vi "Untitled 3.vi"() -> ()   [LabVIEW 2016]
panel:
  out "channel name(s) in (Untitled)":string[](array[string])=["C0", "C1", "C2", "C3", "C4", "C5", "C6", "C7", "C8", "PCR-KW-A", "PCR-KW-B", "PCR-KW-C", "C12", "C13", "C14", "C15", "C16", "C17", "C18", "C19", "C20", "C21", "C22", "", "", ""]
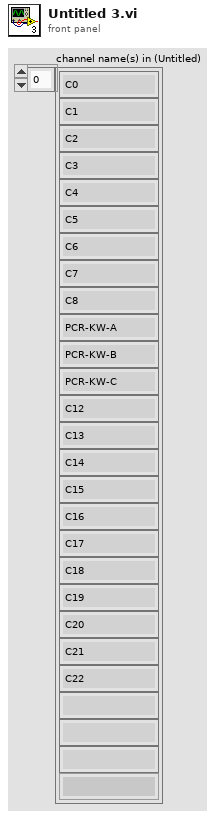
[diagram p1: front panel]
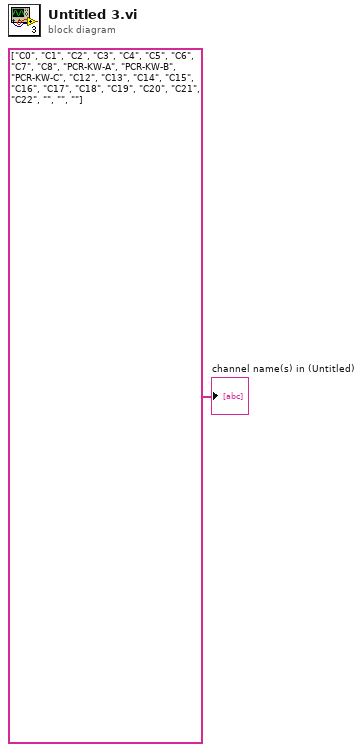
[diagram p0: block diagram]
diagram:
  "channel name(s) in (Untitled)" <- string[] ["C0", "C1", "C2", "C3", "C4", "C5", "C6", "C7", "C8", "PCR-KW-A", "PCR-KW-B", "PCR-KW-C", "C12", "C13", "C14", "C15", "C16", "C17", "C18", "C19", "C20", "C21", "C22", "", "", ""] ("channel name(s) in (Untitled)")
